vi "Write Data Bus.vi"(8 "error in (no error)":errorcluster, 10 "Data":u8 format="%02x", 11 "IO in":refnum<class "IO.lvclass">) -> (0 "error out":errorcluster, 3 "IO out":refnum<class "IO.lvclass">)   [LabVIEW 2021, in "IO.lvclass"]
uses:
  IO.lvclass
  IO.lvclass/IO.ctl
  <vilib>/DAQmx/write.llb/DAQmx Write (Digital 1D Bool NChan 1Samp 1Line).vi
  <vilib>/DAQmx/miscellaneous.llb/DAQmx Fill In Error Info.vi
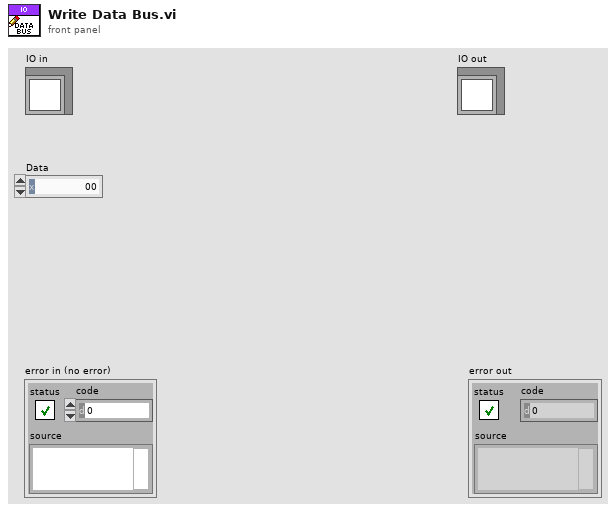
[diagram p1: front panel]
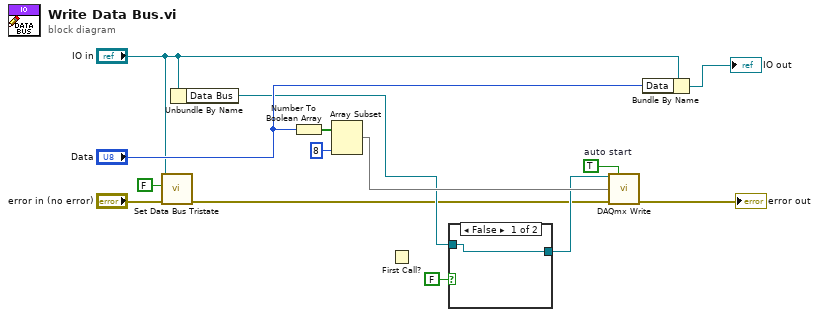
[diagram p0: block diagram]
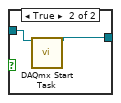
[diagram p2: hidden frame]
diagram:
  w14 = TRUE  # auto start
  n1 = call "Set Data Bus Tristate.vi"("error in (no error)"="error in (no error)", "Tristate"=FALSE, "IO in"="IO in") -> ("error out"=w1:errorcluster)  [unwired: 7 in, 1 out]
  n2 = Unbundle By Name("IO in") -> ("Data Bus"=w5:refnum<k21>)
  n3 = Number To Boolean Array(number="Data") -> (Boolean array=w12:bool[])
  n4 = Array Subset(array=w12, length=8) -> (w10:bool[])  [unwired: 1 in]
  n5 = First Call?() -> ()  [unwired: 1 out]
  n6 = case shown="False" FALSE {
    tunnel: w5 -> [w15 w17]
    tunnel: [w15 w16] -> w7
    frame False {
    }
    frame True {
      n7 = call <vilib>:"DAQmx Start Task.vi"("task/channels in"=w17) -> ("task out"=w16:refnum<k21>)  [unwired: 13 in, 1 out]
    }
  }
  n8 = call-poly <vilib>:"DAQmx Write.vi"("task/channels in"=w7, "auto start"=w14, "data"=w10, "error in"=w1) -> ("error out"=→"error out":errorcluster)  [unwired: 9 in, 2 out]
  n9 = Bundle By Name(cluster="IO in", "Data"="Data") -> (→"IO out":refnum<class "IO.lvclass">)
